vi "TemperatureRunningAverage.vi"() -> ()   [LabVIEW 2025]
panel:
  out "Waveform Chart":cluster{"number: 0 to 1":dbl, dbl}(graph)
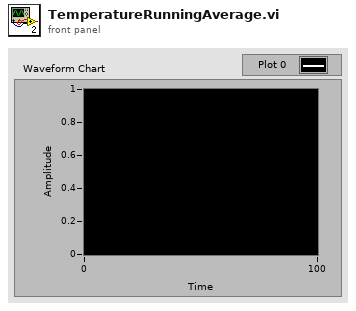
[diagram p1: front panel]
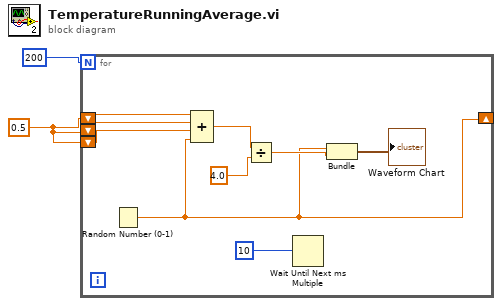
[diagram p0: block diagram]
diagram:
  w1 = 0.5
  n1 = for {
    N: 200 -> [_]
    shift-right: [w5] -> _
    shift-left: w1 -> [w11]
    shift-left: w1 -> [w10]
    shift-left: w1 -> [w9]
    n2 = Random Number (0-1)() -> (number: 0 to 1=w5:dbl)
    n3 = Compound Arithmetic op=ADD(w11, w10, w9, w5) -> (w7:dbl)
    n4 = Divide(x=w7, y=4.0) -> (x/y=w6:dbl)
    n5 = Wait Until Next ms Multiple(millisecond multiple=10) -> ()  [unwired: 1 out]
    n6 = Bundle("number: 0 to 1"=w5, w6) -> (→"Waveform Chart":cluster{"number: 0 to 1":dbl, dbl})  [unwired: 1 in]
  }
